vi "Vessel().vi"() -> (0 "error out":errorcluster, 3 "Vessel.lvclass":refnum<class "Vessel.lvclass">)   [LabVIEW 2014, in "Vessel.lvclass"]
uses:
  Vessel.lvclass
  Thrust Allocation/Thrust Allocation().vi
  Controller/Joystick Controller/Joystick Controller().vi
  Thrust Allocation/Thrust Allocation.lvclass
  Controller/Joystick Controller/Joystick Controller.lvclass
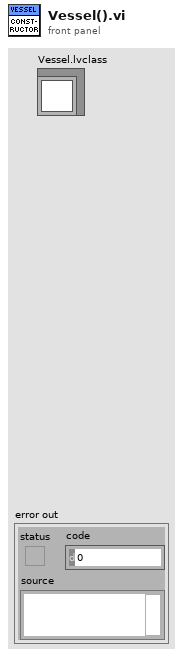
[diagram p1: front panel]
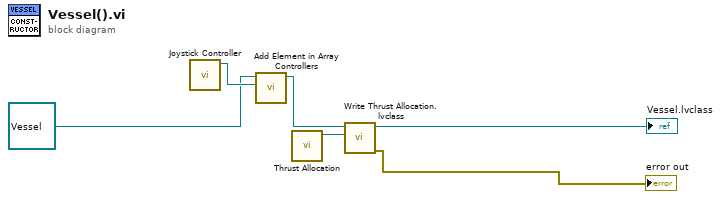
[diagram p0: block diagram]
diagram:
  n1 = call-poly "Joystick Controller.vi"() -> ("Joystick Controller Out"=w4:refnum<class "Joystick Controller.lvclass">)  [unwired: 11 in]
  n2 = call "Add Element in Array Controllers.vi"("Controller Input"=w4, "Vessel in"=refnum<class "Vessel.lvclass"> refnum ("Vessel.lvclass")) -> ("Vessel out"=w2:refnum<class "Vessel.lvclass">)  [unwired: 7 in, 2 out]
  n3 = call-poly "Thrust Allocation.vi"() -> ("Thrust Allocation Out"=w6:refnum<class "Thrust Allocation.lvclass">)  [unwired: 11 in]
  n4 = call "Write Thrust Allocation.lvclass.vi"("Thrust Allocation.lvclass"=w6, "Vessel in"=w2) -> ("error out"=→"error out":errorcluster, "Vessel out"=→"Vessel.lvclass":refnum<class "Vessel.lvclass">)  [unwired: 8 in]
